vi "Cal BC (Numeric).vi"(8 "error in (no error)":errorcluster, 10 "BC in":variant, 11 "Domain_Evolut_2D_Rect in":refnum<class "NI_Domain_Evolut_2D_Rect.lvclass">) -> (0 "error out":errorcluster, 2 "BC out":variant, 3 "Domain_Evolut_2D_Rect out":refnum<class "NI_Domain_Evolut_2D_Rect.lvclass">)   [LabVIEW 2020, in "NI_PDE.lvlib" / "NI_Domain_Evolut_2D_Rect.lvclass"]
uses:
  <vilib>/gmath/pde.llb/DomainClass/Domain_Evolut_2D_Rect/NI_Domain_Evolut_2D_Rect.lvclass
  <vilib>/gmath/pde.llb/BCClass/BC_Evolut_2D_Numeric/BC Data.ctl
  <vilib>/gmath/pde.llb/Common/PDE_BC Type.ctl
  <vilib>/gmath/pde.llb/Common/PDE_BC Position 2D.ctl
  <vilib>/gmath/pde.llb/DomainClass/Domain_Evolut_2D_Rect/NI_Domain_Evolut_2D_Rect.lvclass/NI_Domain_Evolut_2D_Rect.ctl
  <vilib>/gmath/NI_PDE.lvlib
  <vilib>/gmath/pde.llb/BCClass/BC_Evolut_2D_Numeric/NI_BC_Evolut_2D_Numeric.lvclass
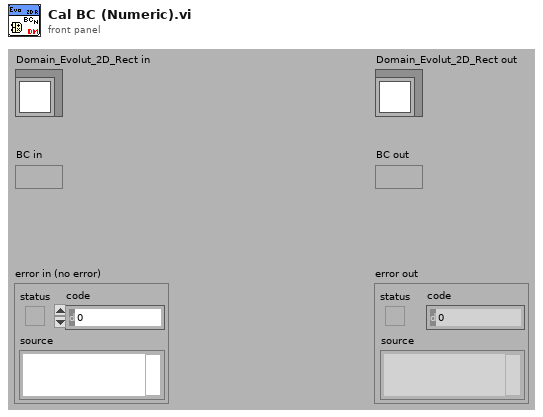
[diagram p1: front panel]
types:
  T1 = typedef "NI_PDE.lvlib/NI_BC_Evolut_2D_Numeric.lvclass/BC Data.ctl" = cluster{"type":T2, "position":T3, "G":dbl[][]}
  T2 = typedef "NI_PDE.lvlib/PDE_BC Type.ctl" = i32
  T3 = typedef "NI_PDE.lvlib/PDE_BC Position 2D.ctl" = i32
  T4 = cluster{"initial t":dbl, "final t":dbl, "# of t-points":i32}
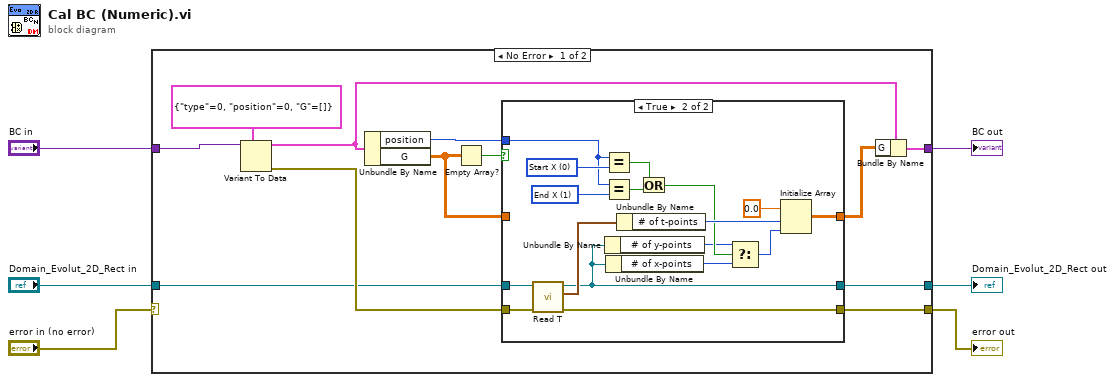
[diagram p0: block diagram]
diagram:
  n1 = case shown="No Error" "error in (no error)" {
    selector: "error in (no error)" -> [_ w41]
    tunnel: "Domain_Evolut_2D_Rect in" -> [w10 w40]
    tunnel: [w7 w40] -> w6
    tunnel: [w8 w41] -> w5
    tunnel: [w16 w39] -> w2
    tunnel: "BC in" -> [w18 w39]
    frame No Error {
      n2 = Variant To Data(type=T1 {"type"=0, "position"=0, "G"=[]} ("BC data"), Variant=w18) -> (data=w13:T1, error out=w11:errorcluster)  [unwired: 1 in]
      n3 = Unbundle By Name(w13) -> ("position"=w12:T3, "G"=w15:dbl[][])
      n4 = Empty Array?(array=w15) -> (empty?=w14:bool)
      n5 = case shown="True" w14 {
        tunnel: w10 -> [w19 w24]
        tunnel: w11 -> [w20 w23]
        tunnel: w15 -> [w21 _]
        tunnel: [w20 w35] -> w8
        tunnel: [w21 w37] -> w9
        tunnel: w12 -> [_ w25]
        tunnel: [w19 w22] -> w7
        frame False {
        }
        frame True {
          w32 = T3 1 items=["Start X", "End X", "Start Y", "End Y"] ("y")
          w33 = T3 0 items=["Start X", "End X", "Start Y", "End Y"] ("y")
          n6 = call-dynamic "Read T.vi"("error in (no error)"=w23, "Domain_Evolut.lvclass in"=w24) -> ("error out"=w35:errorcluster, "t"=w38:T4, "Domain_Evolut.lvclass out"=w22:refnum<class "NI_Domain_Evolut_2D_Rect.lvclass">)  [unwired: 7 out]
          n7 = Equal?(x=w25, y=w33) -> (x = y?=w31:bool)
          n8 = Equal?(x=w25, y=w32) -> (x = y?=w30:bool)
          n9 = Unbundle By Name(w22) -> ("# of y-points"=w28:i32)
          n10 = Unbundle By Name(w22) -> ("# of x-points"=w27:i32)
          n11 = Unbundle By Name(w38) -> ("# of t-points"=w34:i32)
          n12 = Or(x=w31, y=w30) -> (x .or. y?=w29:bool)
          n13 = Select(t=w28, s=w29, f=w27) -> (s? t:f=w26:i32)
          n14 = Initialize Array(0.0 ("element"), w34, w26) -> (w37:dbl[][])
        }
      }
      n15 = Bundle By Name(cluster=w13, "G"=w9) -> (w16:T1)
    }
    frame Error {
    }
  }
  "Domain_Evolut_2D_Rect out" <- w6
  "error out" <- w5
  "BC out" <- w2
